vi "CreateFolders.vi"(8 "error in (no error)":errorcluster, 11 "Messages in":T1[](array[typedef])) -> (0 "error out":errorcluster, 3 "Messages out":T1[](array[typedef]))   [LabVIEW 2017, in "MessageGen.lvlib"]
uses:
  <vilib>/addons/InsightCM/MessageBus/CodeGen/MessageGen.lvlib
  <vilib>/addons/InsightCM/MessageBus/CodeGen/controls/MessageData.ctl
  <vilib>/addons/InsightCM/MessageBus/CodeGen/controls/MessageType.ctl
  <vilib>/addons/InsightCM/MessageBus/CodeGen/controls/Parameter.ctl
  <vilib>/addons/InsightCM/MessageBus/CodeGen/controls/ParameterType.ctl
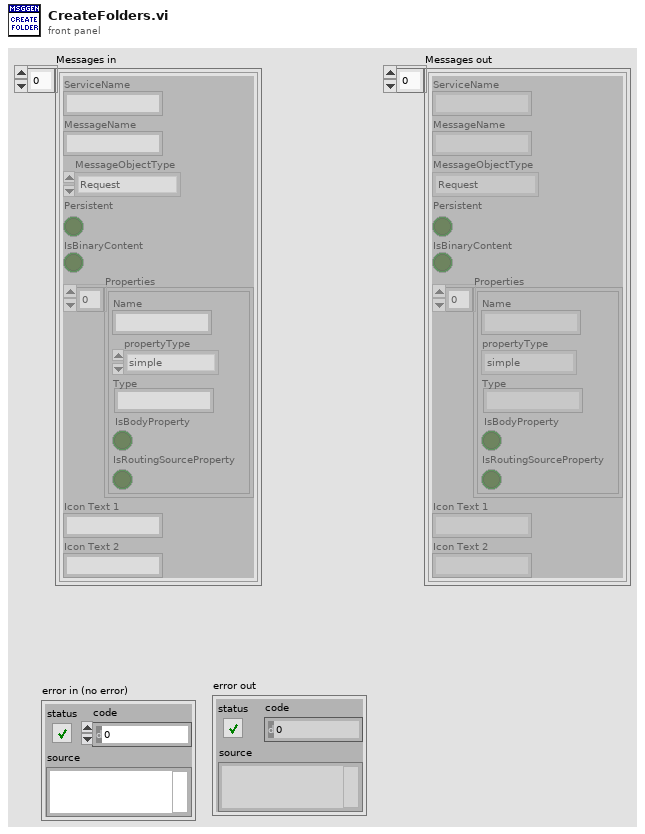
[diagram p1: front panel]
types:
  T1 = typedef "MessageGen.lvlib/MessageData.ctl" = cluster{"ServiceName":string, "MessageName":string, "MessageObjectType":T2, "Persistent":bool, "IsBinaryContent":bool, "Properties":T3[], "Icon Text 1":string, "Icon Text 2":string}
  T2 = typedef "MessageGen.lvlib/MessageType.ctl" = enum16{"Request", "Response", "Broadcast", "RoutedMessage"}
  T3 = typedef "MessageGen.lvlib/Parameter.ctl" = cluster{"Name":string, "propertyType":T4, "Type":string, "IsBodyProperty":bool, "IsRoutingSourceProperty":bool}
  T4 = typedef "MessageGen.lvlib/ParameterType.ctl" = enum16{"simple", "bytearray", "dateTime", "list", "map", "object"}
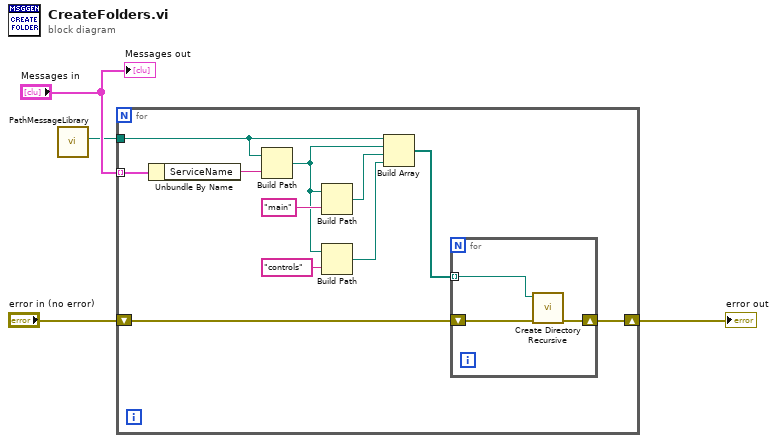
[diagram p0: block diagram]
diagram:
  n1 = call <vilib>:"PathMessageLibrary.vi"() -> ("Path"=w1:path)  [unwired: 11 in]
  n2 = for {
    shift-right: [w14] -> w3
    shift-left: "error in (no error)" -> [w15]
    tunnel: "Messages in" -> [w12] mode=indexing
    tunnel: w1 -> [w9]
    n3 = Unbundle By Name(w12) -> ("ServiceName"=w11:string)
    n4 = Build Path(base path=w9, name or relative path=w11) -> (appended path=w7:path)
    n5 = Build Path(base path=w7, name or relative path="main") -> (appended path=w6:path)
    n6 = Build Path(base path=w7, name or relative path="controls") -> (appended path=w5:path)
    n7 = Build Array(w9, w7, w6, w5) -> (w13:path[])
    n8 = for {
      shift-right: [w17] -> w14
      shift-left: w15 -> [w18]
      tunnel: w13 -> [w16] mode=indexing
      n9 = call <vilib>:"Create Directory Recursive.vi"("error in (no error)"=w18, "directory"=w16) -> ("error out"=w17:errorcluster)  [unwired: 3 in, 2 out]
    }
  }
  "error out" <- w3
  "Messages out" <- "Messages in"
